vi "Test Comm.vi"() -> ()   [LabVIEW 2021]
uses:
  ChannelCommon/typedef/FIFO Config.ctl
  ChannelCommon/ChannelCommon.lvlib
  CIFChannels/Typedef/Direction.ctl
  CIFChannels/CIFChannels.lvclass
  FIFO_DAQ/CIF_NIChn_FIFO_DAQ.lvclass
  ChannelCommon/typedef/TimeStamps.ctl
  D:/dev/Packages/Channel_Manager/src/CIF_NIChn/FIFO_U8/CIF_NIChn_Fifo_U8.lvclass
  D:/dev/Packages/Channel_Manager/src/CIF_NIChn/NIChn/CIF_NIChn.lvclass
  D:/dev/Packages/Channel_Manager/src/CIFChannels/CIFChannels.lvclass
  D:/dev/Packages/Channel_Manager/src/CIF_NIChn/Archive/FIFO_DAQ/CIF_NIChn_FIFO_DAQ.lvclass
  ChannelCommon/typedef/Datatype Waveform.ctl
panel:
  out "Array":errorcluster[](array[cluster])
  out "status":string
  out "pass":bool
  out "error out":errorcluster
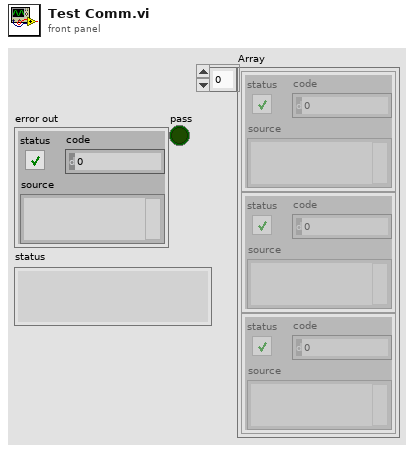
[diagram p1: front panel]
types:
  T1 = typedef "CIFChannels.lvclass/Direction.ctl" = enum16{"Publisher", "Subscriber"}
  T2 = typedef "ChannelCommon.lvlib/TimeStamps.ctl" = cluster{"ClockID":u8, "T0":i64, "T_Out":i64}
  T3 = typedef "ChannelCommon.lvlib/FIFO Config.ctl" = cluster{"Max Bytes/Msg":u64, "Max Msg/FIFO":u64, "Flags":u64}
  T4 = typedef "ChannelCommon.lvlib/Datatype Waveform.ctl" = cluster{"measurement":dbl[], "dT":dbl, "Timestamp":i64, "Read Lock":bool}
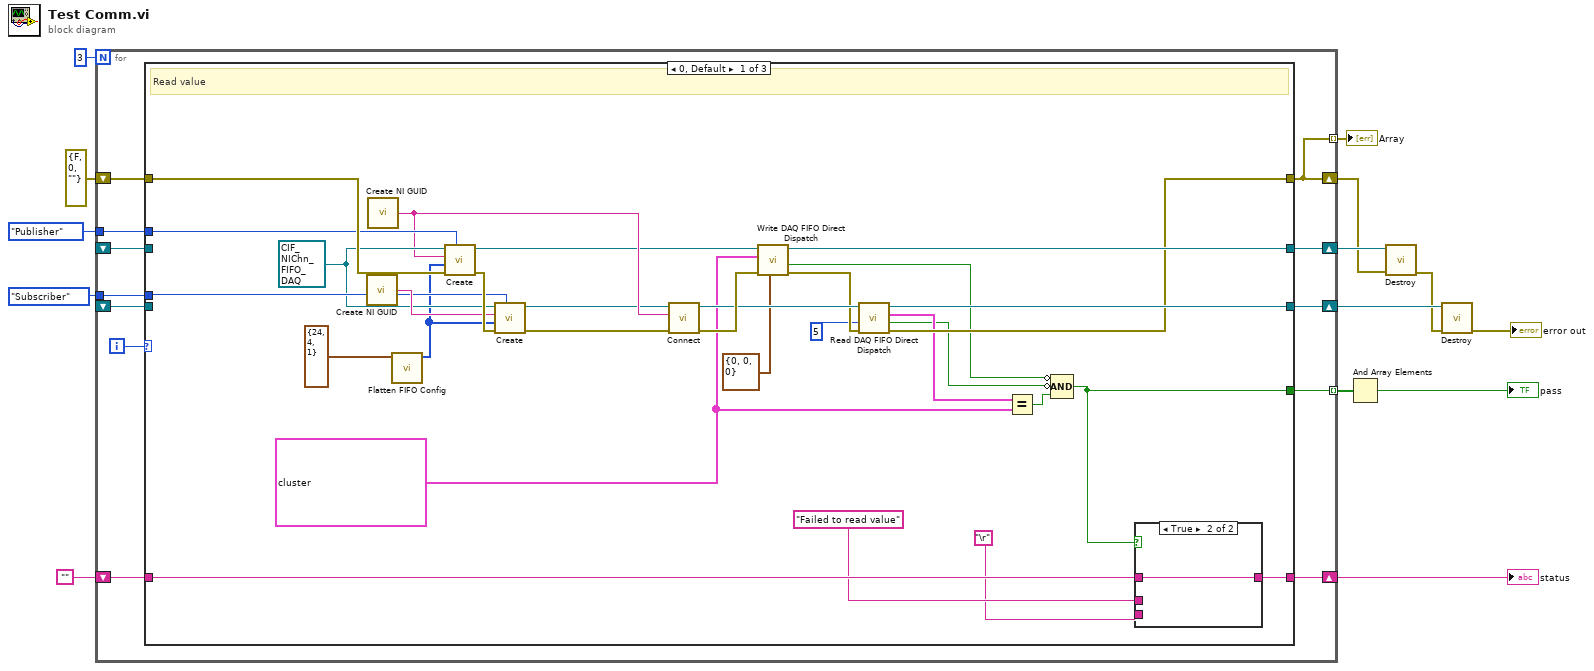
[diagram p0: block diagram]
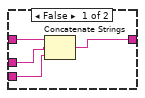
[diagram p2: hidden frame]
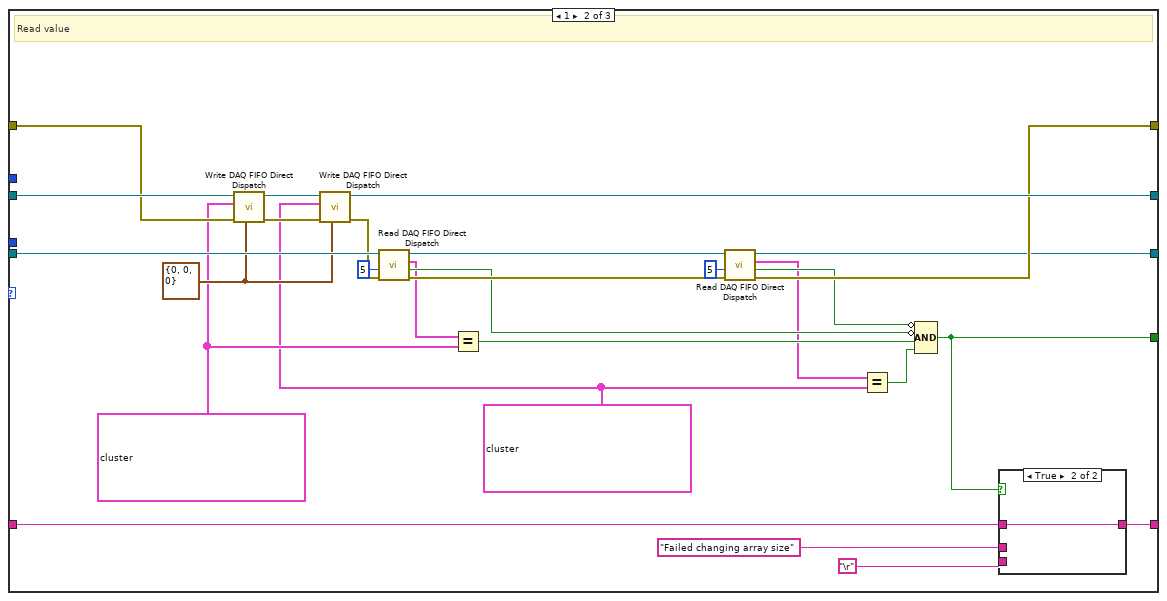
[diagram p3: hidden frame]
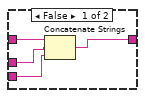
[diagram p4: hidden frame]
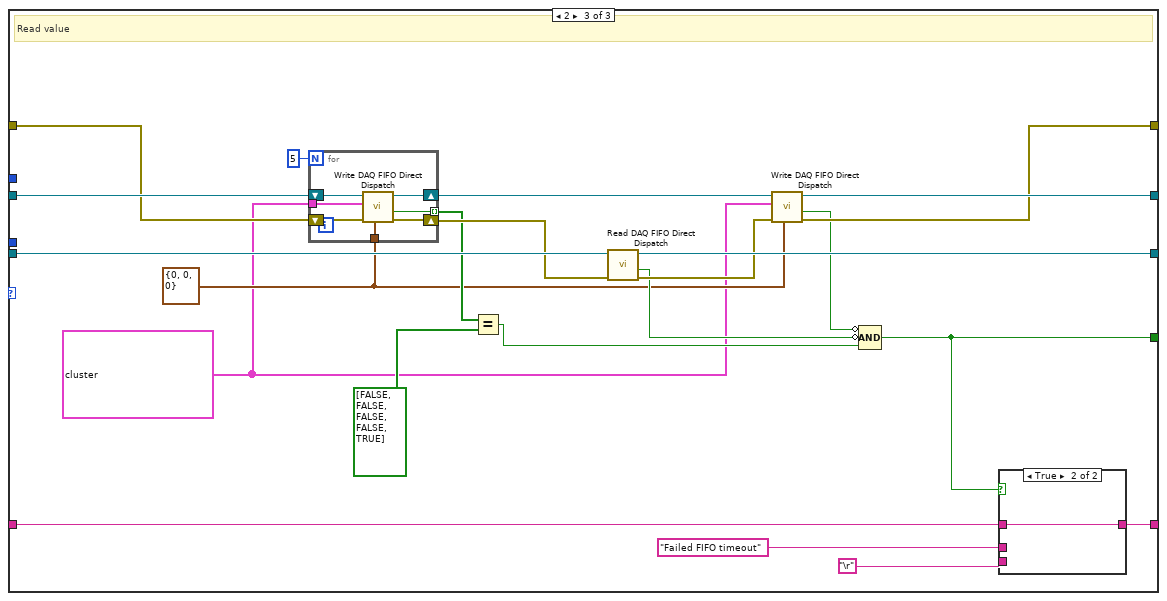
[diagram p5: hidden frame]
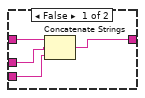
[diagram p6: hidden frame]
diagram:
  n1 = for {
    N: 3 -> [_]
    tunnel: [w26] -> w14 mode=indexing
    shift-right: [w15] -> w4
    shift-left: errorcluster {"status"=FALSE, "code"=0, "source"=""} ("error out") -> [w25]
    shift-right: [w22] -> w10
    shift-left: "" -> [w23]
    tunnel: Direction."Subscriber" ("Direction") -> [w21]
    tunnel: Direction."Publisher" ("Direction") -> [w20]
    shift-right: [w19] -> w6
    shift-left: _ -> [w17]
    shift-right: [w18] -> w5
    shift-left: _ -> [w16]
    tunnel: [w15] -> w1 mode=indexing
    i -> [w24]
    n2 = case shown="0, Default" w24 {
      tunnel: [w51 w84 w96] -> w26
      tunnel: w25 -> [w49 w80 w110]
      tunnel: [w35 w73 w102] -> w15
      tunnel: w23 -> [w56 w88 w115]
      tunnel: [w55 w87 w114] -> w22
      tunnel: w21 -> [w47 _ _]
      tunnel: w20 -> [w46 _ _]
      tunnel: [w36 w70 w107] -> w19
      tunnel: [w38 w77 w105] -> w18
      tunnel: w16 -> [_ w81 w111]
      tunnel: w17 -> [_ w76 w108]
      frame 0, Default {
        w28 = T4[] [{"measurement"=array[986 elements], "dT"=43.0, "Timestamp"=2, "Read Lock"=FALSE}, {"measurement"=array[1001 elements], "dT"=34.0, "Timestamp"=1, "Read Lock"=FALSE}] ("DAQ In")
        w45 = refnum<class "CIF_NIChn_FIFO_DAQ.lvclass"> refnum ("CIF_NIChn_Fifo_Power.lvclass")
        # "Read value"
        n3 = call <vilib>:"Create NI GUID.vi"() -> ("NI GUID"=w48:string)
        n4 = call <vilib>:"Create NI GUID.vi"() -> ("NI GUID"=w43:string)
        n5 = call "Flatten FIFO Config.vi"("FIFO Config in"=T3 {"Max Bytes/Msg"=24, "Max Msg/FIFO"=4, "Flags"=1}) -> ("Flattened FIFO Config"=w27:u8[])  [unwired: 10 in]
        n6 = call-dynamic "Create.vi"("Direction"=w46, "error in (no error)"=w49, "Custom Config Data"=w27, "Name"=w43, "CIFFIFO in"=w45) -> ("error out"=w50:errorcluster, "CIFFIFO out"=w40:refnum<class "CIF_NIChn_FIFO_DAQ.lvclass">)  [unwired: 5 in]
        n7 = call-dynamic "Create.vi"("Direction"=w47, "error in (no error)"=w50, "Custom Config Data"=w27, "Name"=w48, "CIFFIFO in"=w45) -> ("error out"=w42:errorcluster, "CIFFIFO out"=w41:refnum<class "CIF_NIChn_FIFO_DAQ.lvclass">)  [unwired: 5 in]
        n8 = call-dynamic "Connect.vi"("error in (no error)"=w42, "Connection Name"=w43, "CIFTag in"=w41) -> ("error out"=w39:errorcluster, "CIFTag out"=w37:refnum<class "CIF_NIChn_FIFO_DAQ.lvclass">)  [unwired: 7 in]
        n9 = call "Write DAQ FIFO Direct Dispatch.vi"("FIFO Timestamps"=T2 {"ClockID"=0, "T0"=0, "T_Out"=0}, "error in (no error)"=w39, "DAQ In"=w28, "CIFTag in"=w40) -> ("error out"=w34:errorcluster, "timed out?"=w33:bool, "CIFTag out"=w38:refnum<class "CIF_NIChn_FIFO_DAQ.lvclass">)  [unwired: 4 in, 1 out]
        n10 = call "Read DAQ FIFO Direct Dispatch.vi"("error in (no error)"=w34, "Timeout (ms)"=5, "CIFTag in"=w37) -> ("error out"=w35:errorcluster, "timed out?"=w31:bool, "DAQ Out"=w32:T4[], "CIFTag out"=w36:refnum<class "CIF_NIChn_FIFO_DAQ.lvclass">)  [unwired: 4 in, 1 out]
        n11 = Equal?(x=w32, y=w28) -> (x = y?=w52:bool)
        n12 = Compound Arithmetic op=AND(invert w33, invert w31, w52) -> (w51:bool)
        n13 = case shown="True" w51 {
          tunnel: w56 -> [w60 w61]
          tunnel: [w57 w61] -> w55
          tunnel: "Failed to read value" -> [w59 _]
          tunnel: "\r" -> [w58 _]
          frame False {
            n14 = Concatenate Strings(w60, w59, w58) -> (w57:string)
          }
          frame True {
          }
        }
      }
      frame 1 {
        w62 = T4[] [{"measurement"=array[986 elements], "dT"=213.0, "Timestamp"=2, "Read Lock"=FALSE}, {"measurement"=array[1001 elements], "dT"=32.0, "Timestamp"=1, "Read Lock"=FALSE}, {"measurement"=array[988 elements], "dT"=123.0, "Timestamp"=4, "Read Lock"=FALSE}] ("DAQ In")
        w63 = T4[] [{"measurement"=array[986 elements], "dT"=1.0, "Timestamp"=2, "Read Lock"=FALSE}, {"measurement"=array[1001 elements], "dT"=83.0, "Timestamp"=1, "Read Lock"=FALSE}, {"measurement"=array[988 elements], "dT"=78.0, "Timestamp"=4, "Read Lock"=FALSE}] ("DAQ In")
        w64 = T2 {"ClockID"=0, "T0"=0, "T_Out"=0} ("FIFO Timestamps")
        # "Read value"
        n15 = call "Write DAQ FIFO Direct Dispatch.vi"("FIFO Timestamps"=w64, "error in (no error)"=w80, "DAQ In"=w63, "CIFTag in"=w81) -> ("error out"=w78:errorcluster, "CIFTag out"=w79:refnum<class "CIF_NIChn_FIFO_DAQ.lvclass">)  [unwired: 4 in, 2 out]
        n16 = call "Write DAQ FIFO Direct Dispatch.vi"("FIFO Timestamps"=w64, "error in (no error)"=w78, "DAQ In"=w62, "CIFTag in"=w79) -> ("error out"=w74:errorcluster, "CIFTag out"=w77:refnum<class "CIF_NIChn_FIFO_DAQ.lvclass">)  [unwired: 4 in, 2 out]
        n17 = call "Read DAQ FIFO Direct Dispatch.vi"("error in (no error)"=w74, "Timeout (ms)"=5, "CIFTag in"=w76) -> ("error out"=w72:errorcluster, "timed out?"=w68:bool, "DAQ Out"=w65:T4[], "CIFTag out"=w69:refnum<class "CIF_NIChn_FIFO_DAQ.lvclass">)  [unwired: 4 in, 1 out]
        n18 = Equal?(x=w65, y=w63) -> (x = y?=w82:bool)
        n19 = call "Read DAQ FIFO Direct Dispatch.vi"("error in (no error)"=w72, "Timeout (ms)"=5, "CIFTag in"=w69) -> ("error out"=w73:errorcluster, "timed out?"=w67:bool, "DAQ Out"=w66:T4[], "CIFTag out"=w70:refnum<class "CIF_NIChn_FIFO_DAQ.lvclass">)  [unwired: 4 in, 1 out]
        n20 = Equal?(x=w66, y=w62) -> (x = y?=w83:bool)
        n21 = Compound Arithmetic op=AND(invert w67, invert w68, w82, w83) -> (w84:bool)
        n22 = case shown="True" w84 {
          tunnel: w88 -> [w92 w93]
          tunnel: [w89 w93] -> w87
          tunnel: "Failed changing array size" -> [w91 _]
          tunnel: "\r" -> [w90 _]
          frame False {
            n23 = Concatenate Strings(w92, w91, w90) -> (w89:string)
          }
          frame True {
          }
        }
      }
      frame 2 {
        w94 = T4[] [{"measurement"=array[986 elements], "dT"=43.0, "Timestamp"=2, "Read Lock"=FALSE}, {"measurement"=array[1001 elements], "dT"=34.0, "Timestamp"=1, "Read Lock"=FALSE}] ("DAQ In")
        w95 = T2 {"ClockID"=0, "T0"=0, "T_Out"=0} ("FIFO Timestamps")
        # "Read value"
        n24 = for {
          N: 5 -> [_]
          tunnel: w94 -> [w120]
          tunnel: w95 -> [w119]
          shift-right: [w118] -> w106
          shift-left: w111 -> [w122]
          tunnel: [w117] -> w101 mode=indexing
          shift-right: [w116] -> w104
          shift-left: w110 -> [w121]
          n25 = call "Write DAQ FIFO Direct Dispatch.vi"("FIFO Timestamps"=w119, "error in (no error)"=w121, "DAQ In"=w120, "CIFTag in"=w122) -> ("error out"=w116:errorcluster, "timed out?"=w117:bool, "CIFTag out"=w118:refnum<class "CIF_NIChn_FIFO_DAQ.lvclass">)  [unwired: 4 in, 1 out]
        }
        n26 = Equal?(x=w101, y=bool[] [FALSE, FALSE, FALSE, FALSE, TRUE]) -> (x = y?=w97:bool)
        n27 = call "Read DAQ FIFO Direct Dispatch.vi"("error in (no error)"=w104, "CIFTag in"=w108) -> ("error out"=w103:errorcluster, "timed out?"=w99:bool, "CIFTag out"=w107:refnum<class "CIF_NIChn_FIFO_DAQ.lvclass">)  [unwired: 5 in, 2 out]
        n28 = call "Write DAQ FIFO Direct Dispatch.vi"("FIFO Timestamps"=w95, "error in (no error)"=w103, "DAQ In"=w94, "CIFTag in"=w106) -> ("error out"=w102:errorcluster, "timed out?"=w98:bool, "CIFTag out"=w105:refnum<class "CIF_NIChn_FIFO_DAQ.lvclass">)  [unwired: 4 in, 1 out]
        n29 = Compound Arithmetic op=AND(invert w98, invert w99, w97) -> (w96:bool)
        n30 = case shown="True" w96 {
          tunnel: w115 -> [w126 w127]
          tunnel: [w123 w127] -> w114
          tunnel: "Failed FIFO timeout" -> [w125 _]
          tunnel: "\r" -> [w124 _]
          frame False {
            n31 = Concatenate Strings(w126, w125, w124) -> (w123:string)
          }
          frame True {
          }
        }
      }
    }
  }
  "status" <- w10
  "Array" <- w1
  n32 = And Array Elements(Boolean array=w14) -> (logical AND=→"pass":bool)
  n33 = call-dynamic "Destroy.vi"("error in (no error)"=w4, "CIFFIFO in"=w5) -> ("error out"=w3:errorcluster)  [unwired: 8 in, 1 out]
  n34 = call-dynamic "Destroy.vi"("error in (no error)"=w3, "CIFFIFO in"=w6) -> ("error out"=→"error out":errorcluster)  [unwired: 8 in, 1 out]
